vi "Process.vi"(8 "error in":errorcluster, 11 "Measurement.IVCurve":refnum<class "Measurement.IVCurve.lvclass">) -> (0 "error out":errorcluster, 3 "Measurement.IVCurve out":refnum<class "Measurement.IVCurve.lvclass">)   [LabVIEW 2017, in "Measurement.IVCurve.lvclass"]
doc: "---------------------------------------------------------------\nJKI State Machine Objects™\nhttp://jki.net/state-machine-objects/\nCopyright (C) 2005-2015, JKI <info@jki.net>\nALL RIGHTS RESERVEDJKI State Machine Objects (SMO) 1.0.0.5\nJKI - JKI\nCopyright (c) 2016, JKI"
uses:
  Measurement.IVCurve.lvclass
  D:/Program Files (x86)/National Instruments/LabVIEW 2017/vi.lib/JKI/JKI SMO/SMO/SMO.lvclass
  D:/upwork/Laser Measurement Tool/Laser/project/Subsystems/Measurement/Measurement.lvclass
  <vilib>/JKI/JKI SMO/SMO/Typedefs/Parent Call--Enum.ctl
  Measurement/Typedefs/Measurement.State--Enum.ctl
  Typedefs/Measurement.IVCurve.State--Enum.ctl
  Typedefs/Vector--Cluster.ctl
  Typedefs/Results--Cluster.ctl
  Typedefs/Measurement.IVCurve.Measured--Data.ctl
  Measurement/Typedefs/PublicEvents--Measurement.Finished.ctl
  Measurement/Typedefs/PublicEvents--Measurement.Initialized.ctl
  Measurement/Typedefs/PublicEvents--Measurement.Escaped.ctl
  <vilib>/Analysis/baseanly.llb/Mean (DBL).vi
  SMU/SMU.lvclass
  D:/upwork/Laser Measurement Tool/Laser/project/Subsystems/MeasuringDevice/MeasuringDevice.lvclass
  Measurement/Measurement.lvclass
  <vilib>/JKI/JKI SMO/SMO/SMO.lvclass
  MeasuringDevice/MeasuringDevice.lvclass
  <vilib>/Analysis/NI_AALBase.lvlib
panel:
  # "Measurement.IVCurve\nProcess.vi"
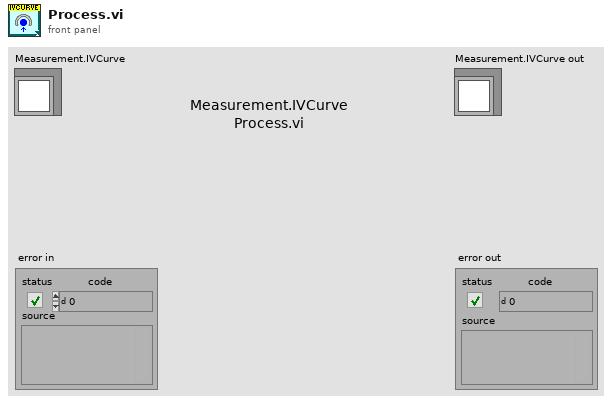
[diagram p1: front panel]
types:
  T1 = typedef "SMO.lvclass/Parent Call--Enum.ctl" = enum16{"Allows parent to run", "Does not request parent to run"}
  T2 = typedef "Measurement.lvclass/Measurement.State--Enum.ctl" = enum16{"Uninitialized", "Initialized", "Started", "Paused", "Stopped"}
  T3 = typedef "Measurement.IVCurve.lvclass/Measurement.IVCurve.State--Enum.ctl" = enum16{"Stoppped", "Wait for Delay time", "Wait for Measurements"}
  T4 = enum32{"invalid app kind", "Development System", "Run Time System", "Student Edition", "Embedded LabVIEW", "Evaluation", "Custom"}
  T5 = enum32{"Invalid", "Standard", "Closed", "Hidden", "Minimized", "Maximized"}
  T6 = typedef "Measurement.lvclass/PublicEvents--Measurement.Finished.ctl" = bool
  T7 = typedef "Measurement.lvclass/PublicEvents--Measurement.Initialized.ctl" = bool
  T8 = typedef "Measurement.IVCurve.lvclass/Dependencies--Cluster.ctl" = cluster{"SMU":refnum<class "SMU.lvclass">}
  T9 = typedef "Measurement.IVCurve.lvclass/Configuration--Cluster.ctl" = cluster{"Measurement.Type":T10, "Hardware":T11, "Measurement":T14}
  T10 = typedef "Measurement.lvclass/Measurement.Type--Enum.ctl" = enum16{"Free", "I/V Curve", "Wavelength sweeping", "Photocurrent mapping"}
  T11 = typedef "Measurement.IVCurve.lvclass/Configuration.Hardware--Cluster.ctl" = cluster{"SMU":T12}
  T12 = typedef "Measurement.lvclass/Configuration.SMU--Cluster.ctl" = cluster{"Enable":bool, "SMU Model":string, "Configuration":T13}
  T13 = typedef "SMU.lvclass/Configuration--Cluster.ctl" = cluster{"VISA Resource":string, "Channel":string}
  T14 = typedef "Measurement.IVCurve.lvclass/Configuration.Measurement--Cluster.ctl" = cluster{"SMU Voltage Start, V":dbl, "SMU Voltage Stop, V":dbl, "SMU Voltage Step, V":dbl, "Delay time, ms":u16, "Accumulation":u16}
  T15 = typedef "Measurement.lvclass/Vector--Cluster.ctl" = cluster{"Values":dbl[], "Index":i32, "Count":i32}
  T16 = typedef "Measurement.IVCurve.lvclass/Results--Cluster.ctl" = cluster{"SMU Completed":bool, "SMU Measurement":dbl}
  T17 = cluster{"Core":cluster{"Current VI Reference":refnum<vi>, "Close Panel on Exit?":bool, "error":errorcluster}, "Self Reference":refnum<class "Measurement.IVCurve.lvclass">, "Dependencies":T8, "Configuration":T9, "Initialized":bool, "Meas State":T2, "IVCurve State":T3, "Next Step":string, "Vector":T15, "Results":T16}
  T18 = cluster{"Current VI Reference":refnum<vi>, "Close Panel on Exit?":bool, "error":errorcluster}
  T19 = typedef "Measurement.IVCurve.lvclass/Measurement.IVCurve.Measured--Data.ctl" = cluster{"Voltage, V":dbl, "Current, A":dbl}
  T20 = typedef "SMO.lvclass/Protected Events.ctl" = cluster{"StopProcesses":refnum<user-event>, "AbortProcesses":refnum<user-event>, "Config Changed":refnum<user-event>, "Dependency":refnum<user-event>}
  T21 = cluster{"Event Registration Refnum":refnum<event-registration>, "Measurement Protected Events":refnum<event-registration>, "SMU Public Events":refnum<event-registration>}
  T22 = typedef "Measurement.lvclass/PublicEvents--Measurement.Escaped.ctl" = bool
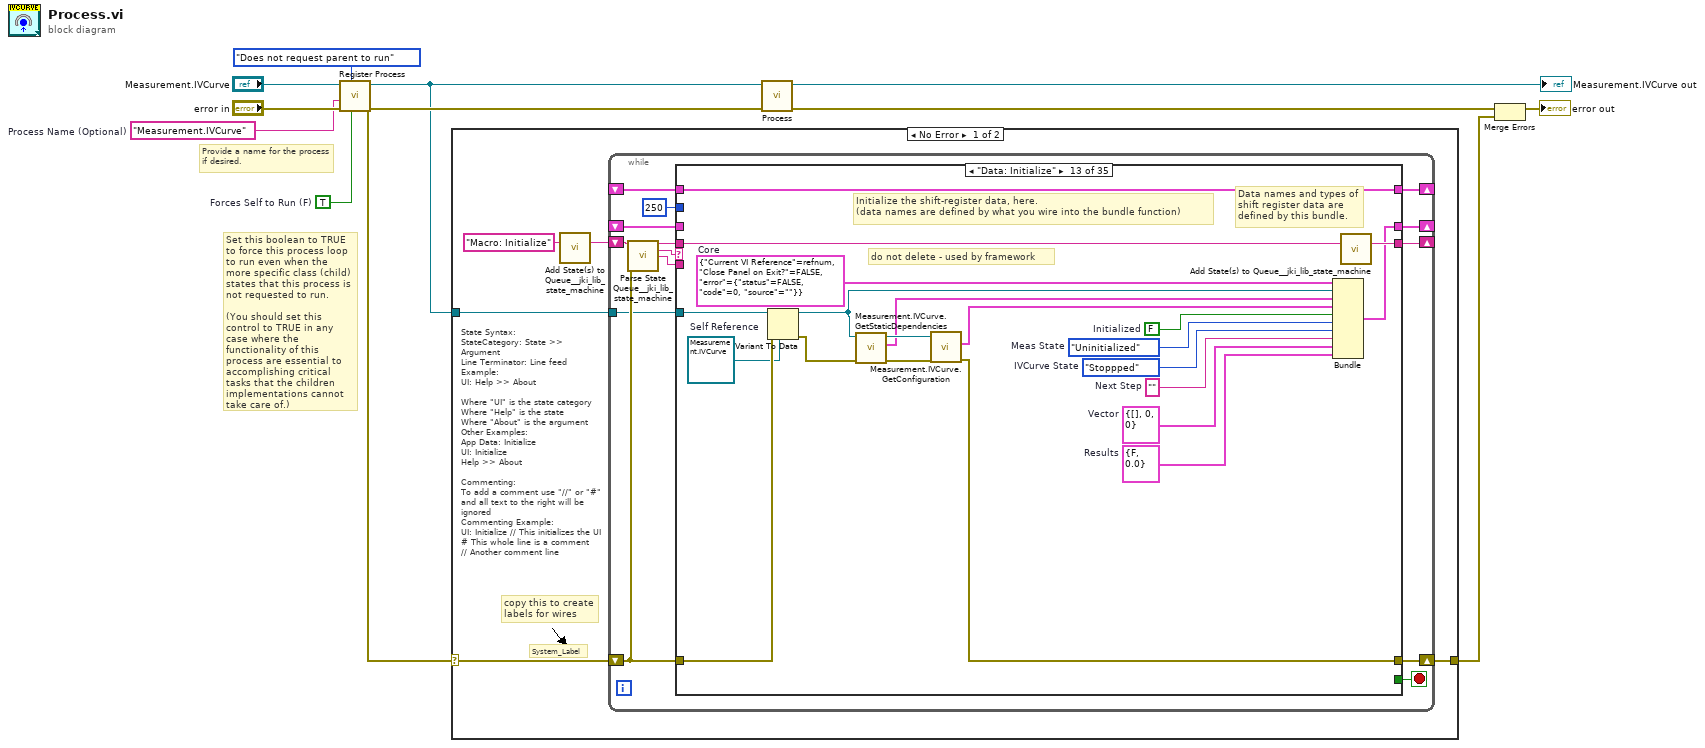
[diagram p0: block diagram]
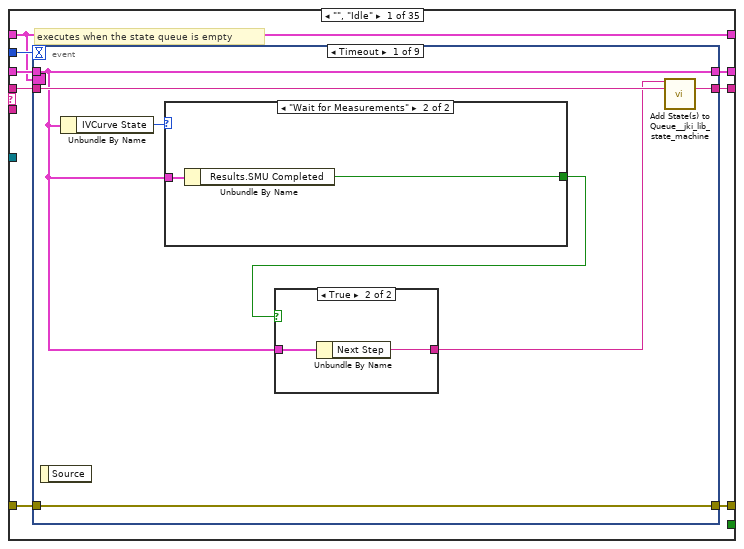
[diagram p2: hidden frame]
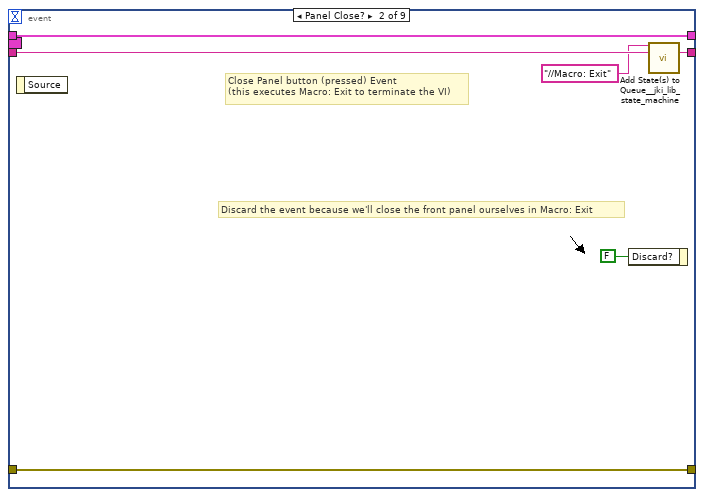
[diagram p5: hidden frame]
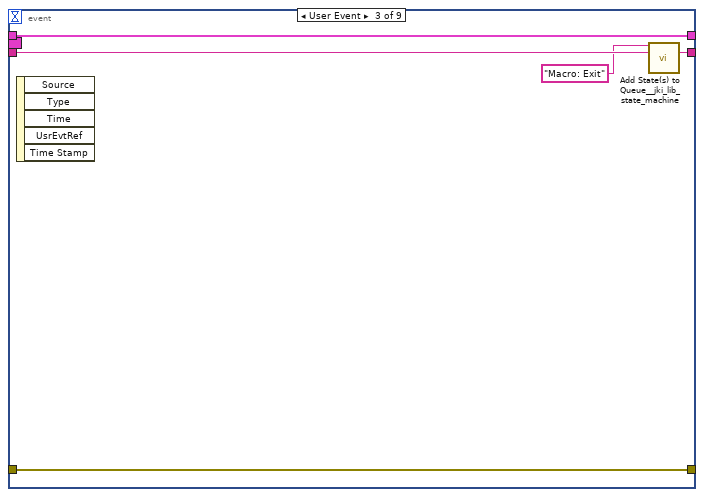
[diagram p6: hidden frame]
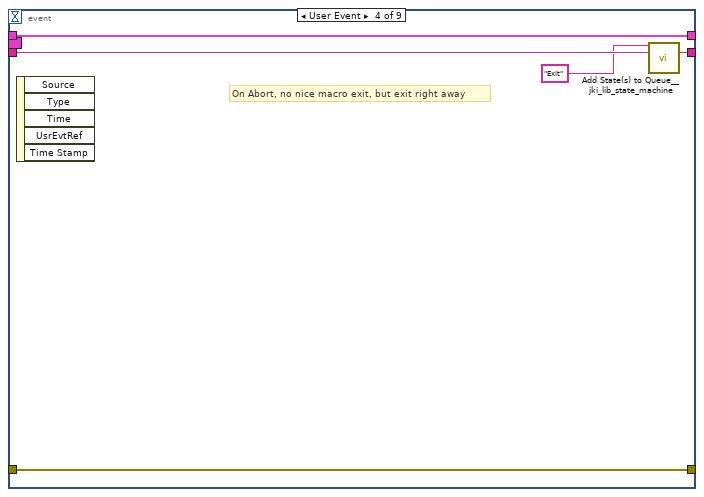
[diagram p7: hidden frame]
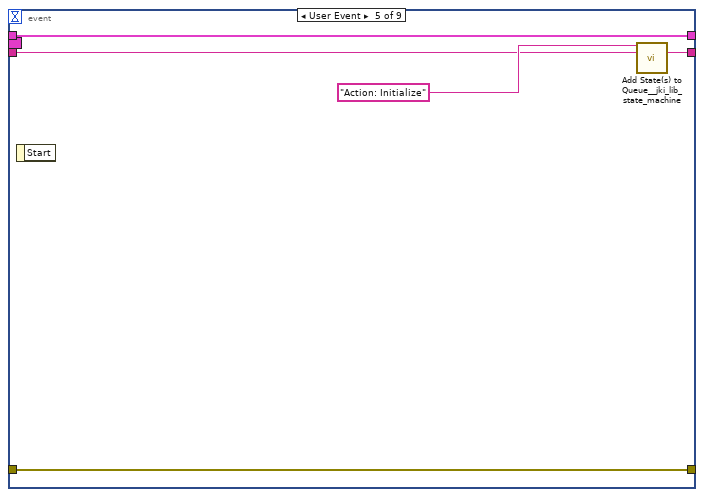
[diagram p8: hidden frame]
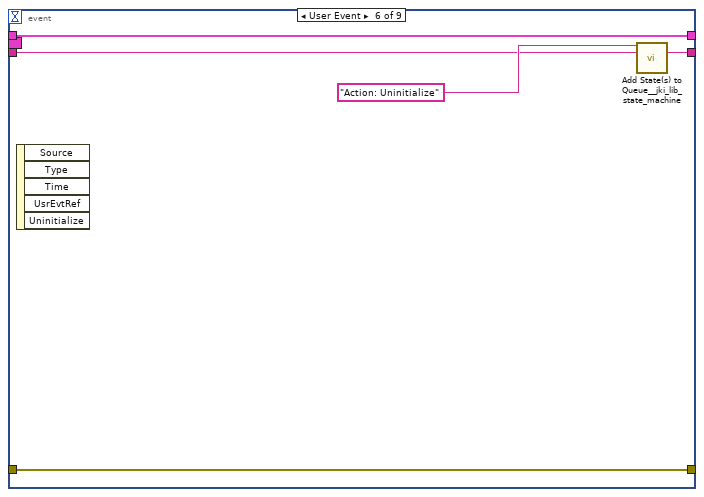
[diagram p9: hidden frame]
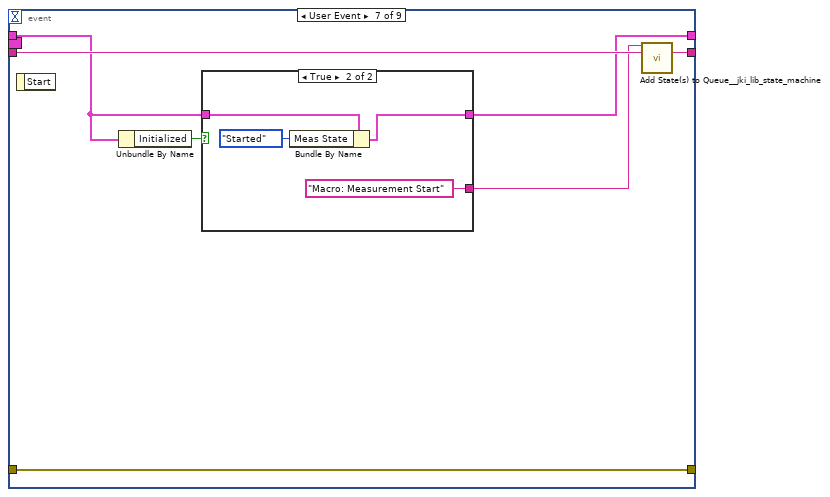
[diagram p10: hidden frame]
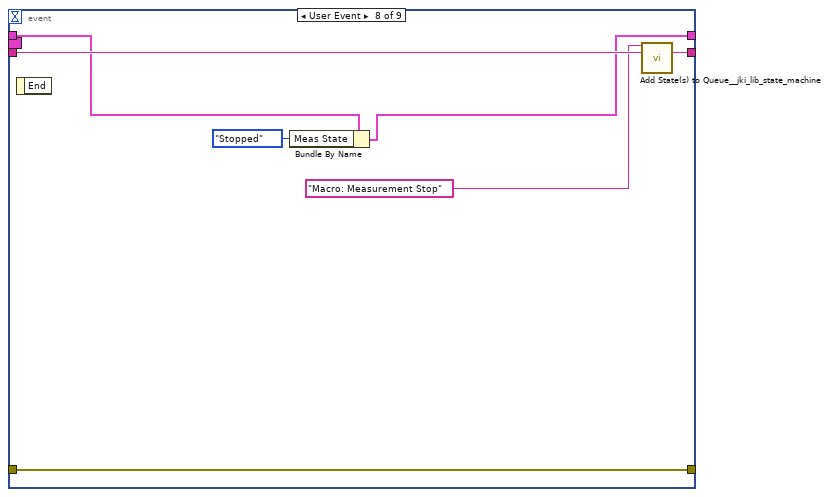
[diagram p12: hidden frame]
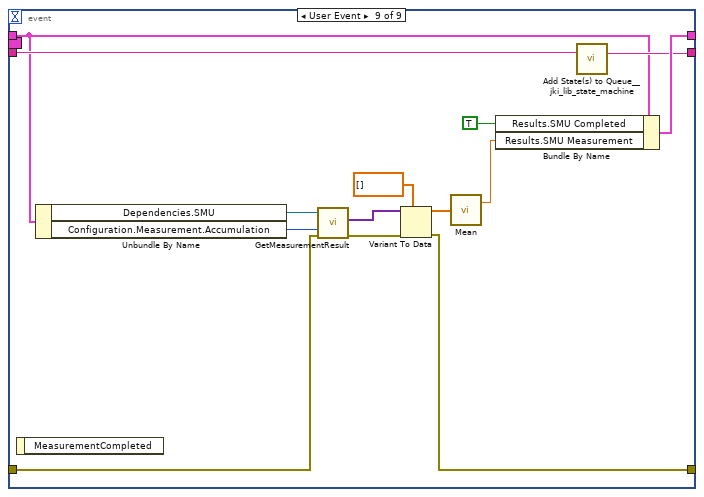
[diagram p13: hidden frame]
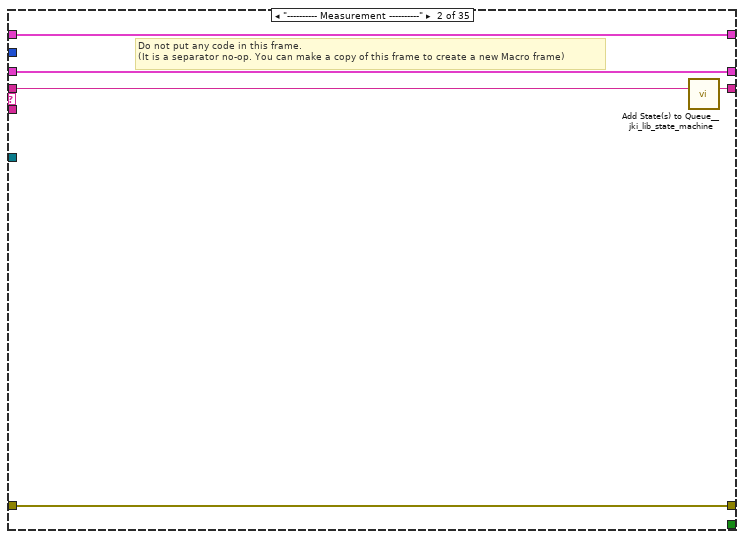
[diagram p14: hidden frame]
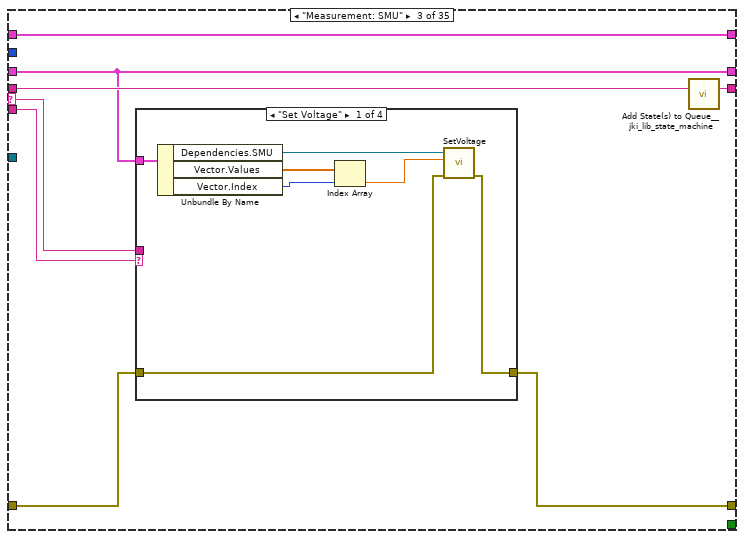
[diagram p15: hidden frame]
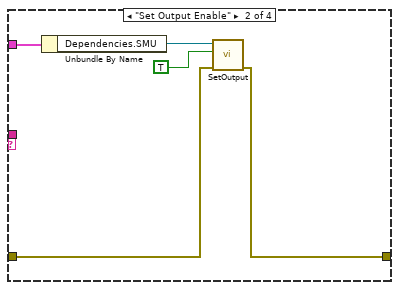
[diagram p16: hidden frame]
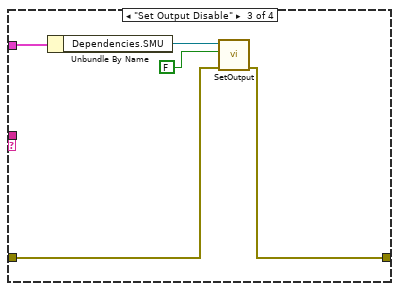
[diagram p17: hidden frame]
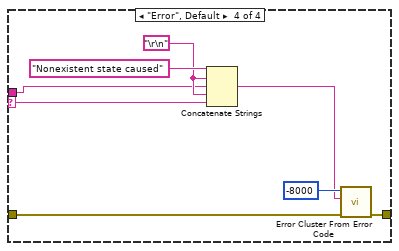
[diagram p18: hidden frame]
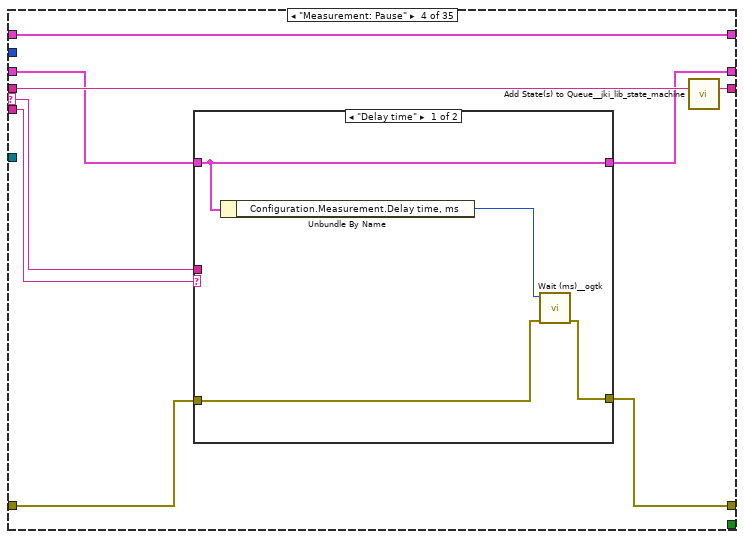
[diagram p19: hidden frame]
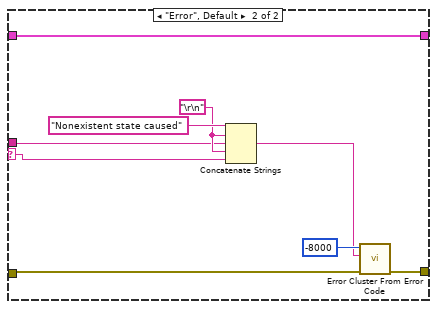
[diagram p20: hidden frame]
diagram:
  w2 = TRUE  # Forces Self to Run (F)
  w1 = "Measurement.IVCurve"  # Process Name (Optional)
  # "Provide a name for the process\nif desired."
  # "Set this boolean to TRUE to force this process loop to run even when the more specific class (child) states that this process is not requested to run.\n\n(You should set this control to TRUE in any case where the functionality of this process are essential to accomplishing critical tasks that the children implementations cannot take care of.)"
  n1 = call <vilib>:"Register Process.vi"("Forces Self to Run (F)"=w2, "Parent Call"=Parent_Call--Enum."Does not request parent to run", "error in (no error)"="error in", "Process Name (optional)"=w1, "SMO"="Measurement.IVCurve") -> ("error out"=w8:errorcluster, "SMO out"=w7:refnum<class "Measurement.IVCurve.lvclass">)  [unwired: 5 in]
  n2 = case shown="No Error" w8 {
    selector: w8 -> [w13 w533]
    tunnel: w7 -> [w14 _]
    tunnel: [w12 w533] -> w4
    frame No Error {
      # "State Syntax:\nStateCategory: State >> Argument\nLine Terminator: Line feed\nExample:\nUI: Help >> About\n\nWhere \"UI\" is the state category\nWhere \"Help\" is the state\nWhere \"About\" is the argument\nOther Examples:\nApp Data: Initialize\nUI: Initialize\nHelp >> About\n\nCommenting:\nTo add a comment use \"//\" or \"#\" and all text to the right will be ignored\nCommenting Example:\nUI: Initialize // This initializes the UI\n# This whole line is a comment\n// Another comment line"
      # "copy this to create labels for wires"
      # "System_Label"
      n3 = call <vilib>:"Add State(s) to Queue__jki_lib_state_machine.vi"("State(s) in (\"\")"="Macro: Initialize") -> ("States Out"=w16:string)  [unwired: 14 in]
      n4 = while {
        shift-right: [w23] -> _
        shift-left: _ -> [w22]
        shift-right: [w26] -> w12
        shift-left: w13 -> [w20]
        shift-right: [w25] -> _
        shift-left: w16 -> [w27]
        tunnel: w14 -> [w19]
        shift-right: [w18] -> _
        shift-left: _ -> [w17]
        stop <- w24 stop-if-true
        n5 = call <vilib>:"Parse State Queue__jki_lib_state_machine.vi"("State Queue"=w27, "Error In (no error)"=w20) -> ("Remaining States"=w29:string, "Current State"=w30:string, "Arguments"=w28:string)  [unwired: 11 in]
        n6 = case shown="\"Data: Initialize\"" w30 {
          selector: w30 -> [_ _ w114 w149 w171 _ _ w222 _ _ _ _ _ _ _ _ _ _ _ _ _ _ _ _ _ _ _ _ _ _ _ _ _ _ _]
          tunnel: w29 -> [w38 w113 w121 w155 w170 w213 w220 w226 w245 w260 w266 w271 w292 w299 w311 w316 w321 w328 w344 w385 w390 w399 w413 w421 w427 w438 w443 w454 w459 w475 w481 w486 w499 w517 w532]
          tunnel: w28 -> [_ _ w119 w152 w176 _ _ _ _ _ _ _ _ _ _ _ _ w322 w338 _ _ _ _ _ _ _ _ _ _ _ _ _ _ _ _]
          tunnel: w22 -> [w36 w110 w117 w151 w173 w205 w217 w224 w236 w250 w262 w268 _ w294 w303 w313 w319 w326 w340 w382 w387 w395 w404 w416 w423 w433 w440 w451 w456 w460 w479 w484 w491 w508 w529]
          tunnel: [w35 w111 w115 w147 w174 w211 w218 w228 w242 w252 w261 w269 w280 w295 w304 w314 w318 w323 w341 w378 w388 w397 w411 w419 w425 w430 w441 w445 w457 w470 w477 w482 w487 w512 w525] -> w26
          tunnel: w20 -> [w34 w111 w116 w148 w175 w211 w218 w227 w242 w247 _ w269 w289 w296 w305 w314 w318 w324 w342 w379 w388 w397 w411 w419 w425 w431 w441 w446 w457 w461 w477 w482 w495 w513 w526]
          tunnel: [w37 w112 w120 w154 w178 w212 w219 w225 w244 w259 w265 w270 w291 w298 w310 w315 w320 w327 w343 w384 w389 w398 w412 w420 w426 w437 w442 w453 w458 w474 w480 w485 w498 w516 w531] -> w25
          tunnel: [_ _ _ _ _ _ _ _ _ _ TRUE _ _ _ _ _ _ _ _ _ _ _ _ _ _ _ _ _ _ _ _ _ _ _ _] -> w24
          tunnel: [w33 w110 w117 w150 w172 w203 w217 w224 w243 w249 w262 w268 w290 w294 w300 w313 w319 w326 w340 w382 w387 w395 w404 w417 w423 w434 w440 w451 w456 w460 w479 w484 w490 w511 w529] -> w23
          tunnel: 250 ("Timeout") -> [w32 _ _ _ _ _ _ _ _ _ _ _ _ _ _ _ _ _ _ _ _ _ _ _ _ _ _ _ _ _ _ _ _ _ _]
          tunnel: w19 -> [_ _ _ _ _ _ _ _ _ _ _ _ w287 _ _ _ _ _ _ _ _ _ _ _ _ _ _ _ _ _ _ _ w496 w514 w528]
          tunnel: [w31 w109 w118 w153 w177 w210 w216 w221 w233 w258 w263 w267 w286 w293 w309 w312 w317 w325 w337 w383 w386 w396 w405 w418 w424 w436 w439 w452 w455 w469 w478 w483 w497 w515 w530] -> w18
          tunnel: w17 -> [w31 w109 w118 w153 w177 w210 w216 w221 w233 w258 w263 w267 w286 w293 w309 w312 w317 w325 w337 w383 w386 w396 w405 w418 w424 w436 w439 w452 w455 _ w478 w483 w497 w515 w530]
          frame "", "Idle" {
            # "executes when the state queue is empty"
            n7 = event shown="[0] Timeout" {
              selector: w31 -> [_ _ _ _ _ _ _ _ _]
              dyn-events: _ -> [_ _ _ _ _ _ _ _ _]
              timeout: w32 -> [_ _ _ _ _ _ _ _ _]
              tunnel: w38 -> [w45 w55 w60 w65 w66 w71 w81 w93 w106]
              tunnel: [w44 w54 w59 w64 w68 w73 w82 w94 w107] -> w37
              tunnel: w36 -> [w40 w52 w57 w62 w69 w74 w77 w90 w105]
              tunnel: [w43 w53 w58 w63 w70 w75 w80 w92 w100] -> w35
              tunnel: w34 -> [w43 w53 w58 w63 w70 w75 w80 w92 w103]
              tunnel: [w40 w52 w57 w62 w69 w74 w76 w89 w108] -> w33
              event Timeout {
                n8 = event-data() -> ()  [unwired: 1 in, 1 out]
                n9 = Unbundle By Name(w40) -> ("IVCurve State"=w42:T3)
                n10 = case shown="\"Wait for Measurements\"" w42 {
                  tunnel: w40 -> [_ w49]
                  tunnel: [_ w48] -> w41
                  frame "Stoppped", Default {
                  }
                  frame "Wait for Measurements" {
                    n11 = Unbundle By Name(w49) -> ("Results.SMU Completed"=w48:bool)
                  }
                }
                n12 = case shown="True" w41 {
                  tunnel: w40 -> [_ w47]
                  tunnel: [_ w46] -> w39
                  frame False {
                  }
                  frame True {
                    n13 = Unbundle By Name(w47) -> ("Next Step"=w46:string)
                  }
                }
                n14 = call <vilib>:"Add State(s) to Queue__jki_lib_state_machine.vi"("State(s) in Front (\"\")"=w39, "State(s) in (\"\")"=w45) -> ("States Out"=w44:string)  [unwired: 13 in]
              }
              event Panel Close? {
                # "Discard the event because we'll close the front panel ourselves in Macro: Exit"
                # "Close Panel button (pressed) Event\n(this executes Macro: Exit to terminate the VI)"
                n15 = event-data() -> ()  [unwired: 1 in, 1 out]
                n16 = event-data("Discard?"=FALSE) -> ()  [unwired: 1 in, 1 out]
                n17 = call <vilib>:"Add State(s) to Queue__jki_lib_state_machine.vi"("State(s) in Front (\"\")"="//Macro: Exit", "State(s) in (\"\")"=w55) -> ("States Out"=w54:string)  [unwired: 13 in]
              }
              event User Event {
                n18 = event-data() -> ()  [unwired: 1 in, 5 out]
                n19 = call <vilib>:"Add State(s) to Queue__jki_lib_state_machine.vi"("State(s) in Front (\"\")"="Macro: Exit", "State(s) in (\"\")"=w60) -> ("States Out"=w59:string)  [unwired: 13 in]
              }
              event User Event {
                # "On Abort, no nice macro exit, but exit right away"
                n20 = event-data() -> ()  [unwired: 1 in, 5 out]
                n21 = call <vilib>:"Add State(s) to Queue__jki_lib_state_machine.vi"("State(s) in Front (\"\")"="Exit", "State(s) in (\"\")"=w65) -> ("States Out"=w64:string)  [unwired: 13 in]
              }
              event User Event {
                n22 = event-data() -> ()  [unwired: 1 in, 1 out]
                n23 = call <vilib>:"Add State(s) to Queue__jki_lib_state_machine.vi"("State(s) in Front (\"\")"="Action: Initialize", "State(s) in (\"\")"=w66) -> ("States Out"=w68:string)  [unwired: 13 in]
              }
              event User Event {
                n24 = event-data() -> ()  [unwired: 1 in, 5 out]
                n25 = call <vilib>:"Add State(s) to Queue__jki_lib_state_machine.vi"("State(s) in Front (\"\")"="Action: Uninitialize", "State(s) in (\"\")"=w71) -> ("States Out"=w73:string)  [unwired: 13 in]
              }
              event User Event {
                n26 = event-data() -> ()  [unwired: 1 in, 1 out]
                n27 = Unbundle By Name(w77) -> ("Initialized"=w78:bool)
                n28 = case shown="True" w78 {
                  tunnel: [_ "Macro: Measurement Start"] -> w79
                  tunnel: w77 -> [w83 w86]
                  tunnel: [w83 w84] -> w76
                  frame False {
                  }
                  frame True {
                    n29 = Bundle By Name(cluster=w86, "Meas State"=Measurement.State--Enum."Started") -> (w84:T17)
                  }
                }
                n30 = call <vilib>:"Add State(s) to Queue__jki_lib_state_machine.vi"("State(s) in Front (\"\")"=w79, "State(s) in (\"\")"=w81) -> ("States Out"=w82:string)  [unwired: 13 in]
              }
              event User Event {
                n31 = event-data() -> ()  [unwired: 1 in, 1 out]
                n32 = Bundle By Name(cluster=w90, "Meas State"=Measurement.State--Enum."Stopped") -> (w89:T17)
                n33 = call <vilib>:"Add State(s) to Queue__jki_lib_state_machine.vi"("State(s) in Front (\"\")"="Macro: Measurement Stop", "State(s) in (\"\")"=w93) -> ("States Out"=w94:string)  [unwired: 13 in]
              }
              event User Event {
                n34 = event-data() -> ()  [unwired: 1 in, 1 out]
                n35 = Unbundle By Name(w105) -> ("Dependencies.SMU"=w104:refnum<class "SMU.lvclass">, "Configuration.Measurement.Accumulation"=w96:u16)
                n36 = call "GetMeasurementResult.vi"("error in (no error)"=w103, "Count (1)"=w96, "MeasuringDevice in"=w104) -> ("error out"=w101:errorcluster, "Result"=w102:variant[])  [unwired: 6 in, 1 out]
                n37 = Variant To Data(error in=w101, type=dbl[] [], Variant=w102) -> (data=w98:dbl[], error out=w100:errorcluster)
                n38 = call-poly <vilib>:"Mean.vi"("X"=w98) -> ("mean"=w97:dbl)  [unwired: 1 out]
                n39 = Bundle By Name(cluster=w105, "Results.SMU Completed"=TRUE, "Results.SMU Measurement"=w97) -> (w108:T17)
                n40 = call <vilib>:"Add State(s) to Queue__jki_lib_state_machine.vi"("State(s) in (\"\")"=w106) -> ("States Out"=w107:string)  [unwired: 14 in]
              }
            }
          }
          frame "---------- Measurement ----------" {
            # "Do not put any code in this frame.\n(It is a separator no-op. You can make a copy of this frame to create a new Macro frame)"
            n41 = call <vilib>:"Add State(s) to Queue__jki_lib_state_machine.vi"("State(s) in (\"\")"=w113) -> ("States Out"=w112:string)  [unwired: 14 in]
          }
          frame "Measurement: SMU" {
            n42 = case shown="\"Set Voltage\"" w119 {
              selector: w119 -> [_ _ _ w140]
              tunnel: w117 -> [w128 w133 w136 _]
              tunnel: w116 -> [w126 w130 w135 w145]
              tunnel: [w125 w129 w134 w144] -> w115
              tunnel: w114 -> [_ _ _ w141]
              frame "Set Voltage" {
                n43 = Unbundle By Name(w128) -> ("Dependencies.SMU"=w127:refnum<class "SMU.lvclass">, "Vector.Values"=w124:dbl[], "Vector.Index"=w123:i32)
                n44 = Index Array(array=w124, index=w123) -> (element=w122:dbl)
                n45 = call "SetVoltage.vi"("error in (no error)"=w126, "Voltage, V"=w122, "SMU in"=w127) -> ("error out"=w125:errorcluster)  [unwired: 7 in, 1 out]
              }
              frame "Set Output Enable" {
                n46 = Unbundle By Name(w133) -> ("Dependencies.SMU"=w132:refnum<class "SMU.lvclass">)
                n47 = call "SetOutput.vi"("error in (no error)"=w130, "Output (False)"=TRUE, "SMU in"=w132) -> ("error out"=w129:errorcluster)  [unwired: 7 in, 1 out]
              }
              frame "Set Output Disable" {
                n48 = Unbundle By Name(w136) -> ("Dependencies.SMU"=w138:refnum<class "SMU.lvclass">)
                n49 = call "SetOutput.vi"("error in (no error)"=w135, "Output (False)"=FALSE, "SMU in"=w138) -> ("error out"=w134:errorcluster)  [unwired: 7 in, 1 out]
              }
              frame "Error", Default {
                w142 = "\r\n"
                n50 = Concatenate Strings("Nonexistent state caused" ("source"), w142, w141, w142, w140) -> (w139:string)
                n51 = call <vilib>:"Error Cluster From Error Code.vi"("error in (no error)"=w145, "error message (\"\")"=w139, "error code (0)"=-8000 ("code")) -> ("error out"=w144:errorcluster)  [unwired: 6 in]
              }
            }
            n52 = call <vilib>:"Add State(s) to Queue__jki_lib_state_machine.vi"("State(s) in (\"\")"=w121) -> ("States Out"=w120:string)  [unwired: 14 in]
          }
          frame "Measurement: Pause" {
            n53 = case shown="\"Delay time\"" w152 {
              selector: w152 -> [_ w160]
              tunnel: w151 -> [w159 w168]
              tunnel: [w159 w168] -> w150
              tunnel: w149 -> [_ w161]
              tunnel: w148 -> [w158 w163]
              tunnel: [w157 w162] -> w147
              frame "Delay time" {
                n54 = Unbundle By Name(w159) -> ("Configuration.Measurement.Delay time, ms"=w156:u16)
                n55 = call <userlib>:"Wait (ms)__ogtk.vi"("error in (no error)"=w158, "milliseconds to wait"=w156) -> ("error out"=w157:errorcluster)  [unwired: 8 in, 1 out]
              }
              frame "Error", Default {
                w165 = "\r\n"
                n56 = Concatenate Strings("Nonexistent state caused" ("source"), w165, w161, w165, w160) -> (w164:string)
                n57 = call <vilib>:"Error Cluster From Error Code.vi"("error in (no error)"=w163, "error message (\"\")"=w164, "error code (0)"=-8000 ("code")) -> ("error out"=w162:errorcluster)  [unwired: 6 in]
              }
            }
            n58 = call <vilib>:"Add State(s) to Queue__jki_lib_state_machine.vi"("State(s) in (\"\")"=w155) -> ("States Out"=w154:string)  [unwired: 14 in]
          }
          frame "Measurement: Measure" {
            n59 = case shown="\"All\"" w176 {
              selector: w176 -> [_ _ w197]
              tunnel: ["Measurement: Measure >> SMU" ("Next Step") w185 w193] -> w169
              tunnel: w175 -> [w183 w191 w196]
              tunnel: [w183 w190 w195] -> w174
              tunnel: w173 -> [w182 w187 w194]
              tunnel: [w181 w189 w194] -> w172
              tunnel: w171 -> [_ _ w198]
              tunnel: w170 -> [w179 w185 w193]
              frame "All" {
                n60 = Bundle By Name(cluster=w182, "IVCurve State"=Measurement.IVCurve.State--Enum."Wait for Measurements" ("W-Sweep State"), "Next Step"=w179) -> (w181:T17)
              }
              frame "SMU" {
                n61 = Unbundle By Name(w187) -> ("Dependencies.SMU"=w192:refnum<class "SMU.lvclass">, "Configuration.Measurement.Accumulation"=w188:u16)
                n62 = Bundle By Name(cluster=w187, "Results.SMU Completed"=FALSE) -> (w189:T17)
                n63 = call "Measure.vi"("error in (no error)"=w191, "Count (1)"=w188, "MeasuringDevice"=w192) -> ("error out"=w190:errorcluster)  [unwired: 6 in, 2 out]
              }
              frame "Error", Default {
                w200 = "\r\n"
                n64 = Concatenate Strings("Nonexistent state caused" ("source"), w200, w198, w200, w197) -> (w199:string)
                n65 = call <vilib>:"Error Cluster From Error Code.vi"("error in (no error)"=w196, "error message (\"\")"=w199, "error code (0)"=-8000 ("code")) -> ("error out"=w195:errorcluster)  [unwired: 6 in]
              }
            }
            n66 = call <vilib>:"Add State(s) to Queue__jki_lib_state_machine.vi"("State(s) in (\"\")"=w169) -> ("States Out"=w178:string)  [unwired: 14 in]
          }
          frame "Measurement: Next Step" {
            n67 = Unbundle By Name(w205) -> ("Vector.Index"=w208:i32, "Vector.Count"=w207:i32)
            n68 = Increment(x=w208) -> (x+1=w204:i32)
            n69 = Less?(x=w204, y=w207) -> (x < y?=w206:bool)
            n70 = case shown="True" w206 {
              tunnel: ["Macro: Measurement Stop" "Macro: Measurement Step"] -> w209
              frame False {
                # "Stop measurement"
              }
              frame True {
                # "1. Do now"
                # "Go to next voltage"
              }
            }
            n71 = Bundle By Name(cluster=w205, "Vector.Index"=w204) -> (w203:T17)
            n72 = call <vilib>:"Add State(s) to Queue__jki_lib_state_machine.vi"("State(s) in Front (\"\")"=w209, "State(s) in (\"\")"=w213) -> ("States Out"=w212:string)  [unwired: 13 in]
          }
          frame "---------- Core ----------" {
            # "Do not put any code in this frame.\n(it is a separator no-op)"
            n73 = call <vilib>:"Add State(s) to Queue__jki_lib_state_machine.vi"("State(s) in (\"\")"=w220) -> ("States Out"=w219:string)  [unwired: 14 in]
          }
          frame Default {
            w231 = 42 items=["No error", "Argument error", "Memory is full", "Out of zone", "End of file", "File already open", "Generic file I/O error", "File not found", "File permission error", "Disk is full", "Duplicate path", "Too many files open", "System feature not enabled", "Resource file not found", "Cannot add resource", "Resource not found", "Image not found", "Image memory error", "Pen does not exist", "Config type invalid", "Config token not found", "Config parse error", "Config memory error", "Bad external code format", "Bad external code offset", "External code not present", "Null window", "Destroy window error", "Null menu", "Print aborted", "Bad print record", "Print driver error", "Windows error during printing", "Memory error during printing", "Print dialog error", "Generic print error", "Invalid device refnum", "Device not found", "Device parameter error", "Device unit error", "Cannot open device", "Device call aborted", "Generic error", "Cancelled by user", "Object ID too low", "Object ID too high", "Object not in heap", "Unknown heap", "Unknown object (invalid DefProc)", "Unknown object (DefProc not in table)", "Message out of range", "Invalid (null) method", "Unknown message", "Manager call not supported", "Bad address", "Network operation in progress", "Network operation timed out", "Connection is busy", "Network attribute not supported", "Network error", "Address in use", "System out of memory", "Connection aborted", "Connection refused", "Not connected", "Already connected", "Connection closed", "Initialization error (interapplication manager)", "Bad occurrence", "Wait on unbound occurrence handler", "Occurrence queue overflow", "Datalog type conflict", "Unused", "Unrecognized type (interapplication manager)", "Memory corrupt", "Failed to make temporary DLL", "Old CIN version", "Drag socket not found", "Failed to load drop-object", "Failed to register OLE object", "Failed to release OLE object", "Format specifier type mismatch", "Unknown format specifier", "Too few format specifiers", "Too many format specifiers", "Scan failed", "Newer CIN version", "Error converting to variant", "Runtime menu error", "Password tampered", "Variant attribute not found", "Incompatible variant data type", "Event data is not available", "Event Store is not present", "Occurrence is not found", "Event Queue is not created", "Event info is not available", "Refnum passed is NULL", "Error retrieving Class GUID", "Error retrieving CoClass GUID", "Error retrieving TypeLib GUID.", "Bad built application magic bytes.", "Specific driver is different from the specific driver associated with the Logical Name.", "There is no session opened to the class driver.", "Max Error", "MAX - Error with config objects", "MAX - Error loading configuration", "MAX - Group not supported"]
            # "Current State"
            # "Do not delete, rename, or modify this frame.\n(this is used to capture unhandled states and typos)"
            # "Handle mistyped state name (developer tool)"
            n74 = Format Into String(format string="Software Exception: Unhandled State \"%s\"." ("message"), error in=w227, w222) -> (resulting string=w230:string, error out=w229:errorcluster)  [unwired: 1 in]
            n75 = call <vilib>:"Error Cluster From Error Code.vi"("show call chain? (False)"=TRUE, "error in (no error)"=w229, "error message (\"\")"=w230, "error code (0)"=w231) -> ("error out"=w228:errorcluster)  [unwired: 5 in]
            n76 = call <vilib>:"Add State(s) to Queue__jki_lib_state_machine.vi"("State(s) in (\"\")"=w226) -> ("States Out"=w225:string)  [unwired: 14 in]
          }
          frame "Initialize Core Data" {
            # "Do not delete, rename, or modify this frame.\n(this is used to determine panel behavior on exit)"
            # "originally closed?"
            # "exe?"
            # "If panel starts closed or is an EXE, then close it when we exit"
            n77 = property class="VI"() -> ("Front Panel.Open"=w241:bool)  [unwired: 2 in, 2 out]
            n78 = property class="App"() -> ("App.Kind"=w240:T4)  [unwired: 2 in, 2 out]
            n79 = control-ref of="Current VI Reference"() -> (w234:refnum<vi>)
            n80 = Not(x=w241) -> (.not. x?=w238:bool)
            n81 = Equal?(x=w240, y=T4."Run Time System" ("Application:Kind")) -> (x = y?=w237:bool)
            n82 = Or(x=w238, y=w237) -> (x .or. y?=w235:bool)
            n83 = Bundle By Name(cluster=w236, "Core.Current VI Reference"=w234, "Core.Close Panel on Exit?"=w235) -> (w243:T17)
            n84 = call <vilib>:"Add State(s) to Queue__jki_lib_state_machine.vi"("State(s) in (\"\")"=w245) -> ("States Out"=w244:string)  [unwired: 14 in]
          }
          frame "Error Handler" {
            w252 = errorcluster {"status"=FALSE, "code"=0, "source"=""}  # No error
            # "Overwrite this method to handle errors and pass to parent if not handled. Parent will fire a public event if the error is not handled up the chain of classes."
            # "Handle any errors here.\nYou can also output any states to clean-up after errors occur"
            n85 = Unbundle By Name(w250) -> ("Self Reference"=w257:refnum<class "Measurement.IVCurve.lvclass">)
            n86 = call <vilib>:"Simple Error Handler.vi"("error in (no error)"=w247) -> ("error out"=w246:errorcluster)  [unwired: 4 in, 4 out]
            n87 = call-dynamic "Handle Error.vi"("Stop on Unhandled Error (T)"=TRUE, "error in"=w246, "Measurement"=w257) -> ("handling error"=w253:errorcluster, "Unhandled error"=w251:errorcluster)  [unwired: 6 in, 1 out]
            n88 = Bundle By Name(cluster=w250, "Core.error"=w251) -> (w249:T17)
            n89 = Select(t="Action: Uninitialize\nAction: Escape", s=w253, f="") -> (s? t:f=w254:string)
            n90 = call <vilib>:"Add State(s) to Queue__jki_lib_state_machine.vi"("State(s) in Front (\"\")"=w254, "State(s) in (\"\")"=w260) -> ("States Out"=w259:string)  [unwired: 13 in]
          }
          frame "Exit" {
            # "Do not put any code in this frame.\n(No errors that occur here will be handled.)"
            n91 = Unbundle By Name(w262) -> ("Core.error"=w261:errorcluster)
            n92 = call <vilib>:"Add State(s) to Queue__jki_lib_state_machine.vi"("State(s) in (\"\")"=w266) -> ("States Out"=w265:string)  [unwired: 14 in]
          }
          frame "---------- Data ----------" {
            # "Do not put any code in this frame.\n(It is a separator no-op. You can make a copy of this frame to create a new Data frame)"
            n93 = call <vilib>:"Add State(s) to Queue__jki_lib_state_machine.vi"("State(s) in (\"\")"=w271) -> ("States Out"=w270:string)  [unwired: 14 in]
          }
          frame "Data: Initialize" {
            w272 = T16 {"SMU Completed"=FALSE, "SMU Measurement"=0.0}  # Results
            w273 = T15 {"Values"=[], "Index"=0, "Count"=0}  # Vector
            w274 = ""  # Next Step
            w275 = Measurement.IVCurve.State--Enum."Stoppped"  # IVCurve State
            w276 = FALSE  # Initialized
            w277 = Measurement.State--Enum."Uninitialized"  # Meas State
            w285 = T18 {"Current VI Reference"=refnum, "Close Panel on Exit?"=FALSE, "error"={"status"=FALSE, "code"=0, "source"=""}}  # Core
            w288 = refnum<class "Measurement.IVCurve.lvclass"> refnum  # Self Reference
            # "do not delete - used by framework"
            # "Data names and types of shift register data are defined by this bundle."
            # "Initialize the shift-register data, here.\n(data names are defined by what you wire into the bundle function)"
            n94 = Variant To Data(error in=w289, type=w288, Variant=w287) -> (data=w284:refnum<class "Measurement.IVCurve.lvclass">, error out=w283:errorcluster)
            n95 = call "Measurement.IVCurve.GetStaticDependencies.vi"("error in (no error)"=w283, "Measurement.IVCurve in"=w284) -> ("error out"=w281:errorcluster, "Dependencies"=w279:T8, "Measurement.IVCurve out"=w282:refnum<class "Measurement.IVCurve.lvclass">)  [unwired: 7 in]
            n96 = call "Measurement.IVCurve.GetConfiguration.vi"("error in (no error)"=w281, "Measurement.IVCurve"=w282) -> ("error out"=w280:errorcluster, "Configuration"=w278:T9)  [unwired: 7 in, 1 out]
            n97 = Bundle("Core"=w285, "Self Reference"=w284, "Dependencies"=w279, "Configuration"=w278, "Initialized"=w276, "Meas State"=w277, "IVCurve State"=w275, "Next Step"=w274, "Vector"=w273, "Results"=w272) -> (w290:T17)  [unwired: 1 in]
            n98 = call <vilib>:"Add State(s) to Queue__jki_lib_state_machine.vi"("State(s) in (\"\")"=w292) -> ("States Out"=w291:string)  [unwired: 14 in]
          }
          frame "Data: Cleanup" {
            # "Cleanup any data and references, here.\n(this is called automatically, by the Macro: Exit)"
            n99 = Unbundle By Name(w294) -> ("Core.Current VI Reference"=w297:refnum<vi>)
            n100 = Close Reference(reference=w297, error in (no error)=w296) -> (error out=w295:errorcluster)
            n101 = call <vilib>:"Add State(s) to Queue__jki_lib_state_machine.vi"("State(s) in (\"\")"=w299) -> ("States Out"=w298:string)  [unwired: 14 in]
          }
          frame "Data: Initialize Vector" {
            n102 = Unbundle By Name(w303) -> ("Configuration.Measurement.SMU Voltage Start, V"=w308:dbl, "Configuration.Measurement.SMU Voltage Stop, V"=w307:dbl, "Configuration.Measurement.SMU Voltage Step, V"=w306:dbl)
            n103 = call "Create Linear Vector.vi"("error in (no error)"=w305, "Step"=w306, "Stop"=w307, "Start"=w308) -> ("error out"=w304:errorcluster, "Count"=w301:i32, "Vector"=w302:dbl[])  [unwired: 5 in]
            n104 = Bundle By Name(cluster=w303, "Vector.Values"=w302, "Vector.Count"=w301) -> (w300:T17)
            n105 = call <vilib>:"Add State(s) to Queue__jki_lib_state_machine.vi"("State(s) in (\"\")"=w311) -> ("States Out"=w310:string)  [unwired: 14 in]
          }
          frame "---------- UI ----------" {
            # "Do not put any code in this frame.\n(It is a separator no-op. You can make a copy of this frame to create a new UI frame)"
            n106 = call <vilib>:"Add State(s) to Queue__jki_lib_state_machine.vi"("State(s) in (\"\")"=w316) -> ("States Out"=w315:string)  [unwired: 14 in]
          }
          frame "UI: Initialize" {
            # "Initialize the User Interface, here.\n(this is called automatically, by the Macro: Init)"
            n107 = call <vilib>:"Add State(s) to Queue__jki_lib_state_machine.vi"("State(s) in (\"\")"=w321) -> ("States Out"=w320:string)  [unwired: 14 in]
          }
          frame "UI: Cursor Set" {
            # "Argument"
            # "Initialize the User Interface, here.\n(this is called automatically, by the Macro: Init)"
            n108 = disable-structure shown="Default" {
              disable-tunnel: w324 -> [w329 w332]
              disable-tunnel: [w329 w331] -> w323
              disable-tunnel: w322 -> [_ w330]
              frame condition #0 {
              }
              frame condition #1 (active) {
                n109 = case shown="\"Busy\"" w330 {
                  tunnel: w332 -> [w334 w336]
                  tunnel: [w333 w335] -> w331
                  frame "Idle", Default {
                    n110 = call <vilib>:"Unset Busy.vi"("error in (no error)"=w334) -> ("error out"=w333:errorcluster)  [unwired: 10 in]
                  }
                  frame "Busy" {
                    n111 = call <vilib>:"Set Busy.vi"("error in (no error)"=w336) -> ("error out"=w335:errorcluster)  [unwired: 9 in, 1 out]
                  }
                }
              }
            }
            n112 = call <vilib>:"Add State(s) to Queue__jki_lib_state_machine.vi"("State(s) in (\"\")"=w328) -> ("States Out"=w327:string)  [unwired: 14 in]
          }
          frame "UI: Front Panel State" {
            # "Argument"
            # "Set Front Panel Open or Closed\n(Usage: \"UI: Front Panel State >> Open|Close\")"
            n113 = Unbundle By Name(w340) -> ("Core.Current VI Reference"=w339:refnum<vi>)
            n114 = disable-structure shown="Default" {
              disable-tunnel: w342 -> [w348 w371]
              disable-tunnel: [w347 w371] -> w341
              disable-tunnel: w339 -> [w346 _]
              disable-tunnel: w338 -> [w345 _]
              frame condition #0 (active) {
                n115 = case shown="\"Open\", Default" w345 {
                  tunnel: w348 -> [w352 w365]
                  tunnel: [w354 w366] -> w347
                  tunnel: w346 -> [w353 w363]
                  frame "Open", Default {
                    n116 = property class="VI"(reference=w353, error in=w352) -> (reference out=w350:refnum<vi>, error out=w351:errorcluster, "FP.State"=w349:T5)
                    n117 = case shown="\"Closed\"" w349 {
                      tunnel: [w357 w360] -> w354
                      tunnel: w351 -> [w356 w360]
                      tunnel: w350 -> [w355 _]
                      frame "Closed" {
                        n118 = invoke class="VI" method="FP.Open"(reference=w355, error in=w356, "Activate"=TRUE, "State"=T5."Standard") -> (error out=w357:errorcluster)  [unwired: 1 in, 4 out]
                      }
                      frame Default {
                      }
                    }
                  }
                  frame "Close" {
                    n119 = property class="VI"(reference=w363, error in=w365) -> (reference out=w362:refnum<vi>, error out=w364:errorcluster, "FP.State"=w361:T5)
                    n120 = case shown="Default" w361 {
                      tunnel: [w367 w370] -> w366
                      tunnel: w364 -> [w367 w369]
                      tunnel: w362 -> [_ w368]
                      frame "Invalid", "Closed" {
                      }
                      frame Default {
                        n121 = invoke class="VI" method="FP.Close"(reference=w368, error in=w369) -> (error out=w370:errorcluster)  [unwired: 1 in, 2 out]
                      }
                    }
                  }
                }
              }
              frame condition #1 {
              }
            }
            n122 = call <vilib>:"Add State(s) to Queue__jki_lib_state_machine.vi"("State(s) in (\"\")"=w344) -> ("States Out"=w343:string)  [unwired: 14 in]
          }
          frame "UI: Send to UI" {
            w376 = T19 {"Voltage, V"=0.0, "Current, A"=0.0}  # Measurement.IVCurve.Measured
            n123 = Unbundle By Name(w382) -> ("Self Reference"=w381:refnum<class "Measurement.IVCurve.lvclass">, "Vector.Values"=w374:dbl[], "Vector.Index"=w373:i32, "Results.SMU Measurement"=w375:dbl)
            n124 = Index Array(array=w374, index=w373) -> (element=w372:dbl)
            n125 = Bundle By Name(cluster=w376, "Voltage, V"=w372, "Current, A"=w375) -> (w380:T19)
            n126 = To Variant(anything=w380) -> (Variant=w377:variant)
            n127 = call "Measurement.OnMeasured.vi"("error in (no error)"=w379, "Payload"=w377, "Measurement in"=w381) -> ("error out"=w378:errorcluster)  [unwired: 7 in, 1 out]
            n128 = call <vilib>:"Add State(s) to Queue__jki_lib_state_machine.vi"("State(s) in (\"\")"=w385) -> ("States Out"=w384:string)  [unwired: 14 in]
          }
          frame "---------- Macro ----------" {
            # "Do not put any code in this frame.\n(It is a separator no-op. You can make a copy of this frame to create a new Macro frame)"
            n129 = call <vilib>:"Add State(s) to Queue__jki_lib_state_machine.vi"("State(s) in (\"\")"=w390) -> ("States Out"=w389:string)  [unwired: 14 in]
          }
          frame "Macro: Initialize" {
            w393 = "UI: Initialize\n//UI: Front Panel State >> Open"  # UI: Initialize //UI: Front Panel State >> Open
            # "Initialization Macro\n(This is called once, when the VI starts)"
            n130 = call <vilib>:"Add State(s) to Queue__jki_lib_state_machine.vi"("State(s) in Front (\"\")"="Data: Initialize\nInitialize Core Data\nEvents: Register\nData: Initialize Vector", "State(s) in (\"\")"="Process: Sync", "State(s) at Back (\"\")"=w393) -> ("States Out"=w392:string)  [unwired: 12 in]
            n131 = call <vilib>:"Add State(s) to Queue__jki_lib_state_machine.vi"("State(s) in Front (\"\")"=w392, "State(s) in (\"\")"=w399) -> ("States Out"=w398:string)  [unwired: 13 in]
          }
          frame "Macro: Exit" {
            # "Exit Macro\n(This is called once, when the VI exits)"
            n132 = Unbundle By Name(w404) -> ("Core.Close Panel on Exit?"=w410:bool)
            n133 = Select(t="UI: Front Panel State >> Close", s=w410, f="") -> (s? t:f=w407:string)
            n134 = call <vilib>:"Add State(s) to Queue__jki_lib_state_machine.vi"("State(s) in Front (\"\")"="Data: Cleanup\nEvents: Unregister", "State(s) in (\"\")"="Process: Sync", "State(s) at Back (\"\")"="Exit") -> ("States Out"=w401:string)  [unwired: 12 in]
            n135 = call <vilib>:"Add State(s) to Queue__jki_lib_state_machine.vi"("State(s) in (\"\")"=w407, "State(s) at Back (\"\")"=w401) -> ("States Out"=w406:string)  [unwired: 13 in]
            n136 = call <vilib>:"Add State(s) to Queue__jki_lib_state_machine.vi"("State(s) in Front (\"\")"=w406, "State(s) in (\"\")"=w413) -> ("States Out"=w412:string)  [unwired: 13 in]
          }
          frame "Macro: Measurement Start" {
            n137 = Bundle By Name(cluster=w416, "Vector.Index"=0) -> (w417:T17)
            n138 = call <vilib>:"Add State(s) to Queue__jki_lib_state_machine.vi"("State(s) in Front (\"\")"="Measurement: SMU >> Set Voltage\nMeasurement: SMU >> Set Output Enable\nMacro: Measurement Step", "State(s) in (\"\")"=w421) -> ("States Out"=w420:string)  [unwired: 13 in]
          }
          frame "Macro: Measurement Step" {
            n139 = call <vilib>:"Add State(s) to Queue__jki_lib_state_machine.vi"("State(s) in Front (\"\")"="Measurement: SMU >> Set Voltage\nMeasurement: Pause >> Delay time\nMeasurement: Measure >> All\nUI: Send to UI\nMeasurement: Next Step", "State(s) in (\"\")"=w427) -> ("States Out"=w426:string)  [unwired: 13 in]
          }
          frame "Macro: Measurement Stop" {
            n140 = Unbundle By Name(w433) -> ("Self Reference"=w432:refnum<class "Measurement.IVCurve.lvclass">)
            n141 = call "Measurement.OnFinished.vi"("error in (no error)"=w431, "Finished"=T6 TRUE, "Measurement in"=w432) -> ("error out"=w430:errorcluster)  [unwired: 7 in, 1 out]
            n142 = Bundle By Name(cluster=w433, "IVCurve State"=Measurement.IVCurve.State--Enum."Stoppped" ("W-Sweep State")) -> (w434:T17)
            n143 = call <vilib>:"Add State(s) to Queue__jki_lib_state_machine.vi"("State(s) in Front (\"\")"="Measurement: SMU >> Set Output Disable", "State(s) in (\"\")"=w438) -> ("States Out"=w437:string)  [unwired: 13 in]
          }
          frame "---------- Process ----------" {
            # "Template Separator\n(You can make a copy of, or modify, this frame)"
            n144 = call <vilib>:"Add State(s) to Queue__jki_lib_state_machine.vi"("State(s) in (\"\")"=w443) -> ("States Out"=w442:string)  [unwired: 14 in]
          }
          frame "Process: Sync" {
            n145 = Unbundle By Name(w451) -> ("Self Reference"=w447:refnum<class "Measurement.IVCurve.lvclass">)
            n146 = call <vilib>:"WaitOnProcessSync.vi"("error in (no error)"=w446, "SMO"=w447) -> ("error out"=w445:errorcluster, "Don't run?"=w450:bool)  [unwired: 7 in, 1 out]
            n147 = Select(t="Data: Cleanup\nEvents: Unregister\nExit", s=w450, f="") -> (s? t:f=w444:string)
            n148 = call <vilib>:"Add State(s) to Queue__jki_lib_state_machine.vi"("State(s) in Front (\"\")"=w444, "State(s) in (\"\")"=w454) -> ("States Out"=w453:string)  [unwired: 13 in]
          }
          frame "---------- Events ----------" {
            # "Template Separator\n(You can make a copy of, or modify, this frame)"
            n149 = call <vilib>:"Add State(s) to Queue__jki_lib_state_machine.vi"("State(s) in (\"\")"=w459) -> ("States Out"=w458:string)  [unwired: 14 in]
          }
          frame "Events: Register" {
            # "Static Dependencies\nPublic Events"
            # "Measurement base\nProtected events"
            # "Base Class Protected Events"
            n150 = Unbundle By Name(w460) -> ("Self Reference"=w467:refnum<class "Measurement.IVCurve.lvclass">)
            n151 = Unbundle By Name(w460) -> ("Dependencies.SMU"=w465:refnum<class "SMU.lvclass">)
            n152 = call "Measurement.GetProtectedEventsRegistration.vi"("Measurement in"=w467) -> ("error out"=w463:errorcluster, "Measurement Protected Events"=w466:refnum<event-registration>)  [unwired: 8 in, 1 out]
            n153 = call <vilib>:"GetProtectedEvents.vi"("SMO"=w467) -> ("error out"=w471:errorcluster, "SMO Protected Events"=w473:T20)  [unwired: 8 in, 1 out]
            n154 = call "SMU.GetPublicEventsRegistration.vi"("SMU"=w465) -> ("error out"=w462:errorcluster, "SMU Public Events"=w464:refnum<event-registration>)  [unwired: 8 in, 1 out]
            n155 = register-events(w473) -> (reference out=w468:refnum<event-registration>, error out=w472:errorcluster)  [unwired: 2 in]
            n156 = Bundle("Event Registration Refnum"=w468, "Measurement Protected Events"=w466, "SMU Public Events"=w464) -> (w469:T21)  [unwired: 1 in]
            n157 = Merge Errors(w472, w471, w463, w462, w461) -> (w470:errorcluster)
            n158 = call <vilib>:"Add State(s) to Queue__jki_lib_state_machine.vi"("State(s) in (\"\")"=w475) -> ("States Out"=w474:string)  [unwired: 14 in]
          }
          frame "Events: Unregister" {
            n159 = Unregister For Events(event registration refnum=w478, error in=w477) -> (error out=w476:errorcluster)
            n160 = call <vilib>:"Clear Errors.vi"("error in (no error)"=w476) -> ()  [unwired: 5 in, 2 out]
            n161 = call <vilib>:"Add State(s) to Queue__jki_lib_state_machine.vi"("State(s) in (\"\")"=w481) -> ("States Out"=w480:string)  [unwired: 14 in]
          }
          frame "---------- API ----------" {
            n162 = call <vilib>:"Add State(s) to Queue__jki_lib_state_machine.vi"("State(s) in (\"\")"=w486) -> ("States Out"=w485:string)  [unwired: 14 in]
          }
          frame "Action: Initialize" {
            n163 = call-dynamic "Measurement.Init.vi"("error in (no error)"=w495, "Measurement.IVCurve in"=w496) -> ("error out"=w494:errorcluster, "Result"=w489:bool, "Measurement.IVCurve out"=w493:refnum<class "Measurement.IVCurve.lvclass">)  [unwired: 6 in, 1 out]
            n164 = case shown="False" w489 {
              tunnel: w494 -> [w503 w506]
              tunnel: [w502 w506] -> w492
              frame False {
                n165 = call <vilib>:"Error Cluster From Error Code.vi"("error in (no error)"=w503, "error message (\"\")"="Measurement Initialization failure" ("source"), "error code (0)"=-8000 ("code")) -> ("error out"=w502:errorcluster)  [unwired: 6 in]
              }
              frame True {
              }
            }
            n166 = call "Measurement.OnInitialized.vi"("error in (no error)"=w492, "Initialized"=w489, "Measurement in"=w493) -> ("error out"=w487:errorcluster)  [unwired: 7 in, 1 out]
            n167 = case shown="True" w489 {
              tunnel: [Measurement.State--Enum."Uninitialized" ("State") Measurement.State--Enum."Initialized" ("State")] -> w488
              frame False {
              }
              frame True {
              }
            }
            n168 = Bundle By Name(cluster=w491, "Meas State"=w488, "Initialized"=w489) -> (w490:T17)
            n169 = call <vilib>:"Add State(s) to Queue__jki_lib_state_machine.vi"("State(s) in (\"\")"=w499) -> ("States Out"=w498:string)  [unwired: 14 in]
          }
          frame "Action: Uninitialize" {
            n170 = Unbundle By Name(w508) -> ("Initialized"=w507:bool)
            n171 = case shown="True" w507 {
              tunnel: w514 -> [_ w524]
              tunnel: w513 -> [w518 w523]
              tunnel: [w518 w520] -> w512
              frame False {
              }
              frame True {
                n172 = call-dynamic "Measurement.Uninit.vi"("error in (no error)"=w523, "Measurement.IVCurve in"=w524) -> ("error out"=w521:errorcluster, "Measurement.IVCurve out"=w522:refnum<class "Measurement.IVCurve.lvclass">)  [unwired: 8 in]
                n173 = call "Measurement.OnUninitialized.vi"("error in (no error)"=w521, "Uninitialized (True)"=T7 TRUE ("Uninitialized"), "Measurement in"=w522) -> ("error out"=w520:errorcluster)  [unwired: 7 in, 1 out]
              }
            }
            n174 = Bundle By Name(cluster=w508, "Initialized"=FALSE, "Meas State"=Measurement.State--Enum."Uninitialized" ("State")) -> (w511:T17)
            n175 = call <vilib>:"Add State(s) to Queue__jki_lib_state_machine.vi"("State(s) in (\"\")"=w517) -> ("States Out"=w516:string)  [unwired: 14 in]
          }
          frame "Action: Escape" {
            w527 = T22 TRUE  # Escaped
            n176 = call "Measurement.OnEscaped.vi"("error in (no error)"=w526, "Escaped"=w527, "Measurement in"=w528) -> ("error out"=w525:errorcluster)  [unwired: 7 in, 1 out]
            n177 = call <vilib>:"Add State(s) to Queue__jki_lib_state_machine.vi"("State(s) in (\"\")"=w532) -> ("States Out"=w531:string)  [unwired: 14 in]
          }
        }
      }
    }
    frame Error {
    }
  }
  n178 = call-parent "Process.vi"("error in"=w8, "SMO"=w7) -> ("error out"=w5:errorcluster, "SMO out"=→"Measurement.IVCurve out":refnum<class "Measurement.IVCurve.lvclass">)  [unwired: 8 in]
  n179 = Merge Errors(w5, w4) -> (→"error out":errorcluster)
